vi "PSK_Mod_Transmit_test_Q.vi"() -> ()   [LabVIEW 2014]
uses:
  <vilib>/addons/Modulation/Analog/controls/Complex Data Waveform.ctl
  <vilib>/addons/Modulation/Digital/General/MT Generate Bits (Galois, PN Order).vi
  <vilib>/addons/Modulation/Digital/Support/Common/Validators/mod_Generate Bits Validate.vi
  <vilib>/addons/Modulation/Analog/support/mod_Set Error Source.vi
  <vilib>/addons/Modulation/Digital/General/subVIs/mod_Generate Bits PN Sequence.vi
  <instrlib>/niUSRP/niUSRP Write Tx Data (CDB Cluster).vi
  <vilib>/addons/Modulation/niDMT.lvlib
  <vilib>/addons/Modulation/niAMT.lvlib
panel:
  out "Antall pakker generert":i32
  out "# elements in queue 1":i32
  out "# elements in queue 2":i32
  out "Antall pakker faktisk sendt":dbl
  out "Number of message bits in burst":i32
  out "After mod":waveform(dbl)(graph)
  out "Tid pakkegen":dbl
  out "Tid modulator":dbl
  out "Tid Sender":dbl
  in  "stop":bool
  in  "Packet Parameters":T1={"Length of sync sequence (20)"=30, "Number of message bits"=128, "Number of guardbits"=40, "PN sequence order (31)"=31, "Number of packets in burst"=30}
  out "Constellation Graph":T2(graph) caption="Tx Signal Constellation"
  out "bits pr burst":i32
  out "input bit stream":i8[](array[numeric]) caption="input package"
  out "time/packet":dbl
  out "error out":errorcluster
  in  "USRP IP address":refnum<k15>="192.168.10.1"
  in  "Tx Parameters":T3={"Tx IQ Sampling\nRate [s/sec]"=400000.0, "Tx Frequency [Hz]"=5795000000.0, "Tx Gain [dB]"=10.0, "Tx Antenna"="TX1"} {"Tx Gain [dB]" format="%#.6p"; "Tx Frequency [Hz]" format="%#.6p"; "Tx IQ Sampling\nRate [s/sec]" format="%#.6p"}
  out "Actual Tx Parameters":T3={"Tx IQ Sampling\nRate [s/sec]"=400000.0, "Tx Frequency [Hz]"=915000000.0, "Tx Gain [dB]"=0.0, "Tx Antenna"="TX1"} {"Tx Gain [dB]" format="%#.6p"; "Tx Frequency [Hz]" format="%#.6p"; "Tx IQ Sampling\nRate [s/sec]" format="%#.6p"}
  in  "filter parameters":T4={"Alpha"=0.5, "Filter Length"=6, "TX Filter"=enum."Root Raised Cos"} {"Alpha" format="%.2f"}
  in  "QPSK System Parameters":T5={"Samples per Symbol"=8, "symbol map"=[], "Differential PSK"=enum."disable", "PSK type"=0, "M-PSK (4)"=4} {"PSK type" items=["normal", "shifted", "offset"]; "symbol map" format="%.3f"}
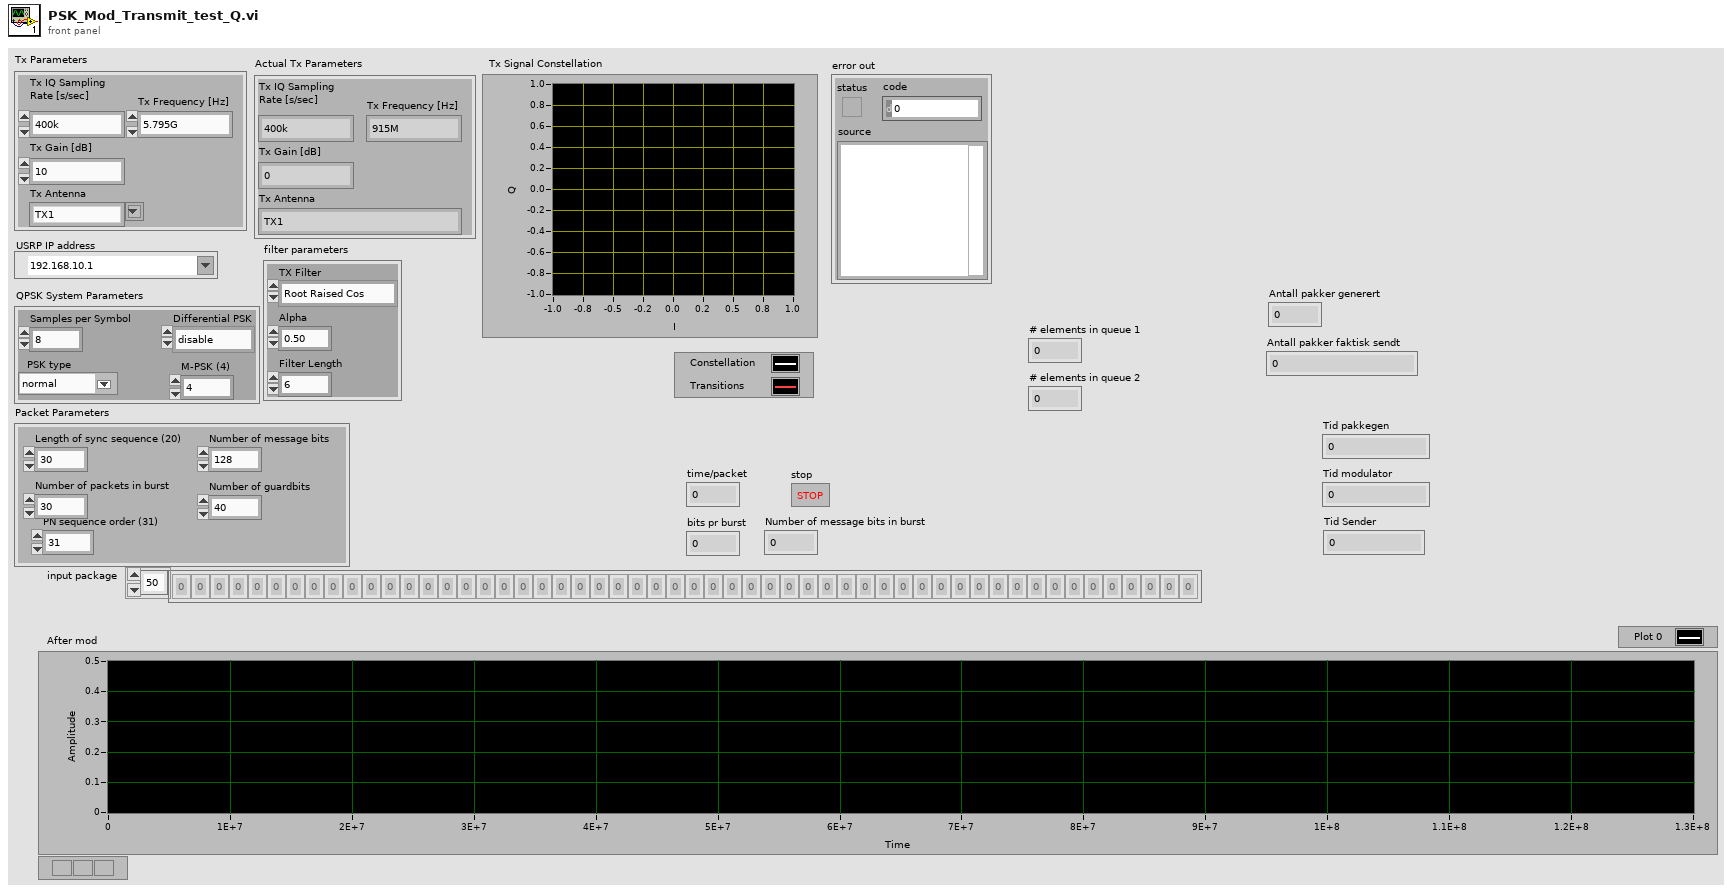
[diagram p1: front panel]
types:
  T1 = cluster{"Length of sync sequence (20)":i32, "Number of message bits":i32, "Number of guardbits":i32, "PN sequence order (31)":i32, "Number of packets in burst":i32}
  T2 = cluster{"constellation":dbl[], "oversampled data":dbl[]}[]
  T3 = cluster{"Tx IQ Sampling\nRate [s/sec]":dbl, "Tx Frequency [Hz]":dbl, "Tx Gain [dB]":dbl, "Tx Antenna":string}
  T4 = cluster{"Alpha":dbl, "Filter Length":i32, "TX Filter":enum16{"none", "Raised Cosine", "Root Raised Cos", "Gaussian"}}
  T5 = cluster{"Samples per Symbol":i32, "symbol map":cdb[], "Differential PSK":enum16{"disable", "enable"}, "PSK type":u16, "M-PSK (4)":i32}
  T6 = typedef "niAMT.lvlib/Complex Data Waveform.ctl" = cluster{"t0":dbl, "dt":dbl, "Y":cdb[]}
  T7 = cluster{"samples per symbol (16)":i32, "symbol map":cdb[], "differential PSK":enum16{"disable", "enable"}, "PSK type":u16}
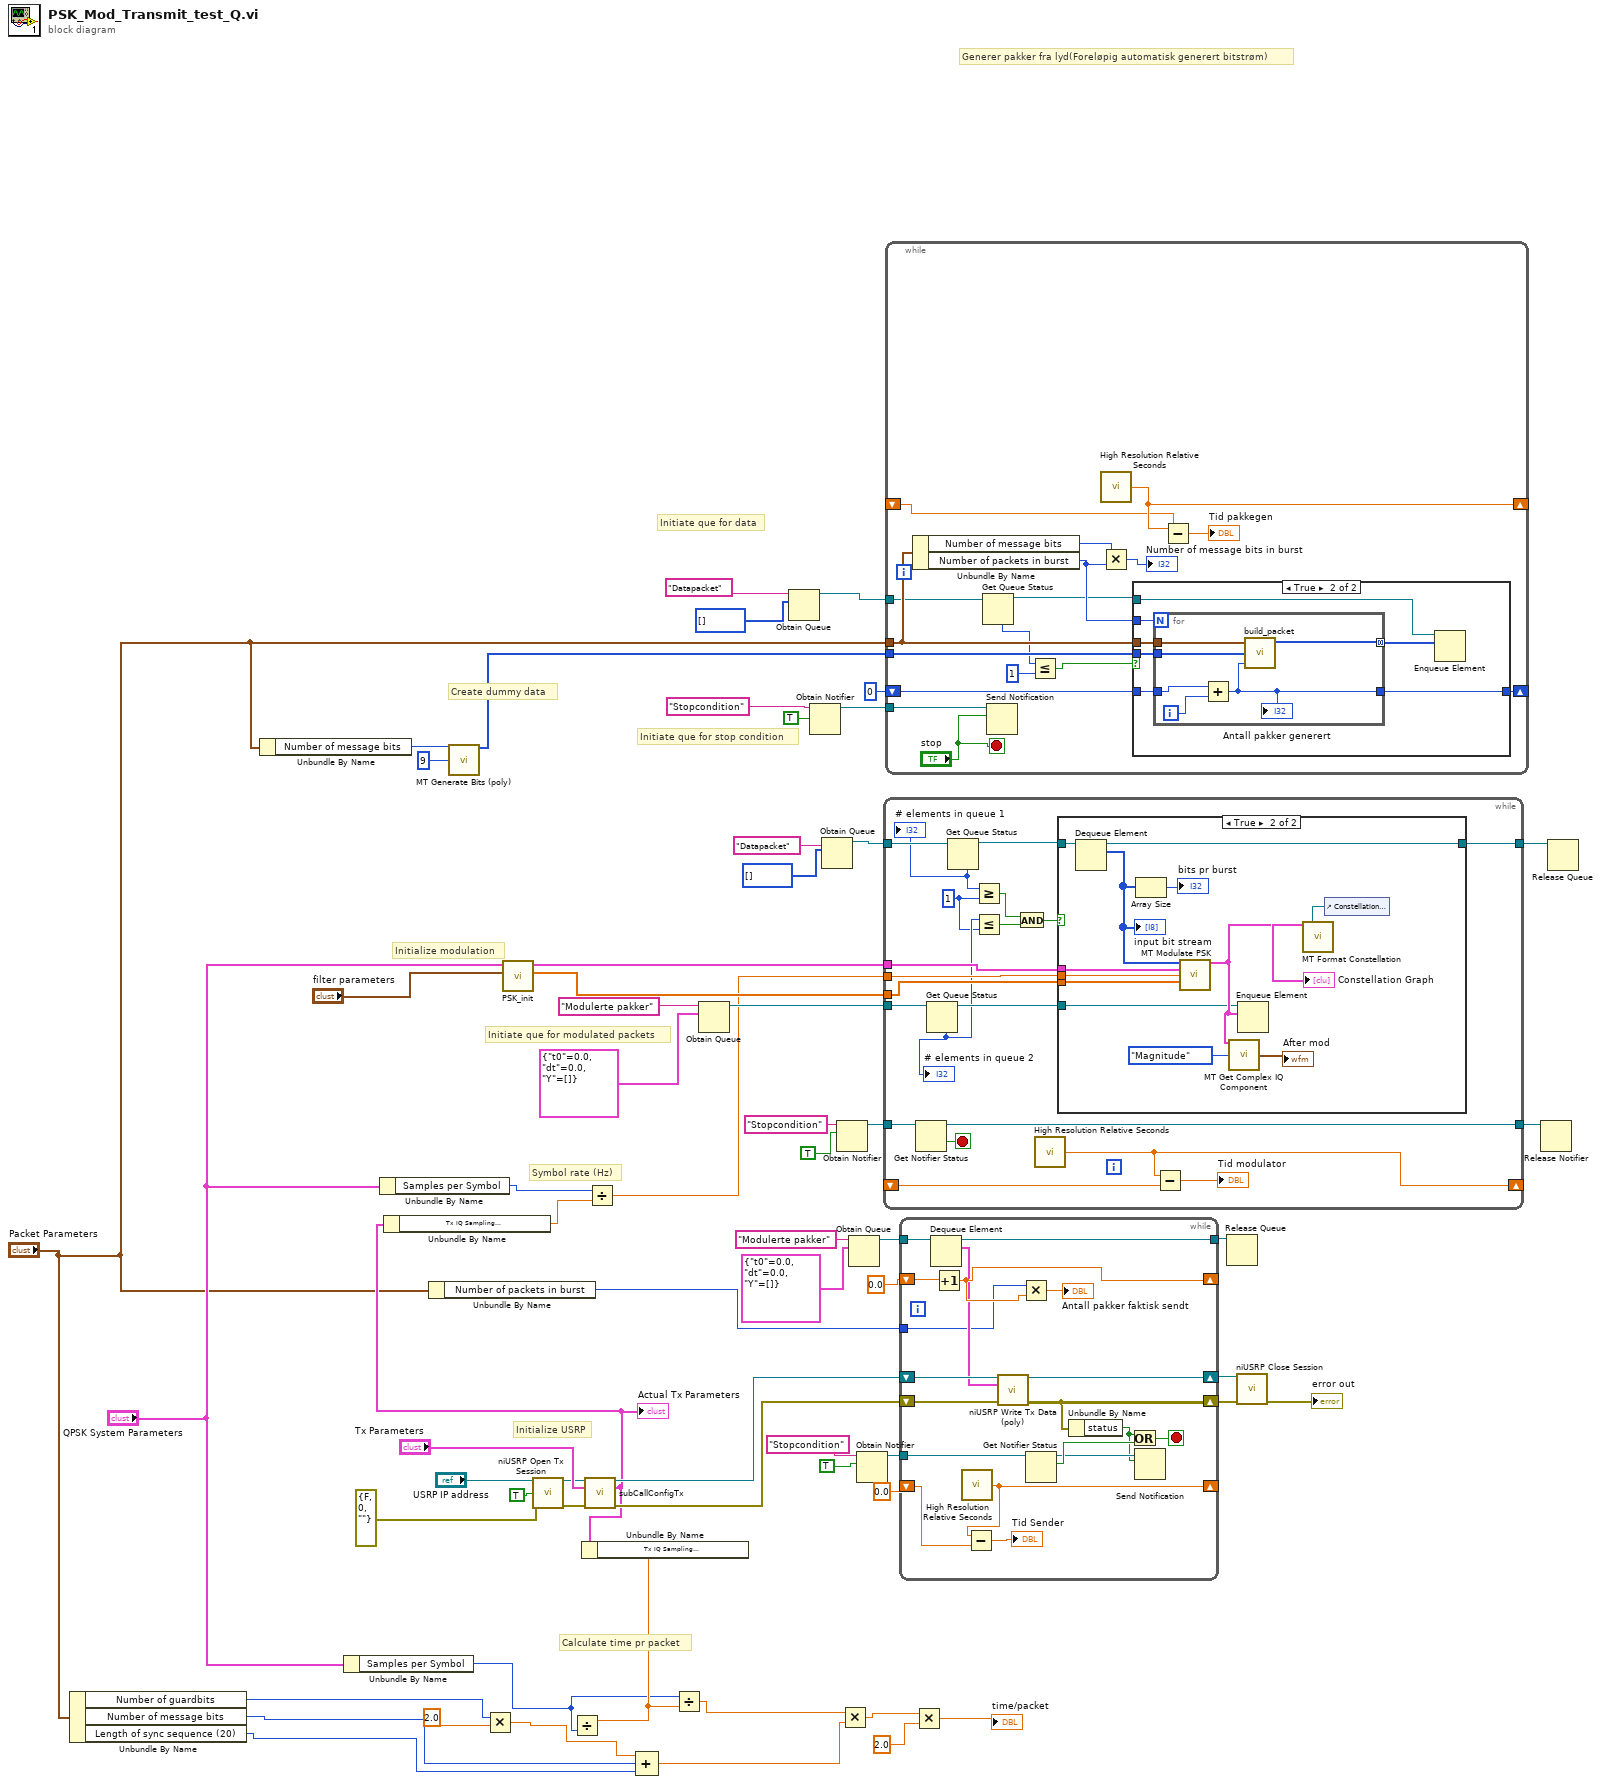
[diagram p0: block diagram]
diagram:
  # "Calculate time pr packet"
  # "Initialize USRP"
  # "Initialize modulation"
  # "Initiate que for modulated packets"
  # "Create dummy data"
  # "Initiate que for stop condition"
  # "Initiate que for data"
  # "Generer pakker fra lyd(Foreløpig automatisk generert bitstrøm)"
  # "Symbol rate (Hz)"
  n1 = Unbundle By Name("Packet Parameters") -> ("Number of guardbits"=w46:i32, "Number of message bits"=w40:i32, "Length of sync sequence (20)"=w44:i32)
  n2 = Unbundle By Name("Packet Parameters") -> ("Number of message bits"=w18:i32)
  n3 = Unbundle By Name("QPSK System Parameters") -> ("Samples per Symbol"=w43:i32)
  n4 = Unbundle By Name("QPSK System Parameters") -> ("Samples per Symbol"=w25:i32)
  n5 = Unbundle By Name("Packet Parameters") -> ("Number of packets in burst"=w2:i32)
  n6 = call-poly <vilib>:"MT Generate Bits (poly).vi"("total bits (128)"=w18, "PN sequence order (9)"=9) -> ("output bit stream"=w19:i8[])  [unwired: 11 in, 2 out]
  n7 = Multiply(x=w46, y=2.0 ("x")) -> (x*y=w53:dbl)
  n8 = call "PSK_init.vi"("filter parameters"="filter parameters", "QPSK System Parameters"="QPSK System Parameters") -> ("matched filter coefficients"=w27:dbl[], "PSK system parameters"=w28:T7)  [unwired: 5 in, 2 out]
  n9 = call <instrlib>:"niUSRP Open Tx Session.vi"("device names"="USRP IP address", "reset"=TRUE, "error in (no error)"=errorcluster {"status"=FALSE, "code"=0, "source"=""}) -> ("session handle out"=w62:refnum<k15>, "error out"=w61:errorcluster)  [unwired: 11 in]
  n10 = call "subCallConfigTx.vi"("session handle"=w62, "Tx Parameters"="Tx Parameters", "error in"=w61) -> ("session handle out"=w57:refnum<k15>, "Actual Tx Parameters"=w21:T3, "error out"=w35:errorcluster)  [unwired: 10 in]
  "Actual Tx Parameters" <- w21
  n11 = Unbundle By Name(w21) -> ("Tx IQ Sampling\nRate [s/sec]"=w24:dbl)
  n12 = Unbundle By Name(w21) -> ("Tx IQ Sampling\nRate [s/sec]"=w52:dbl)
  n13 = Divide(x=w52, y=w43) -> ()  [unwired: 1 out]
  n14 = Divide(x=w25, y=w24) -> (x/y=w23:dbl)
  n15 = Compound Arithmetic op=ADD(w53, w40, w44) -> (w50:dbl)
  n16 = Divide(x=w43, y=w52) -> (x/y=w51:dbl)
  n17 = Obtain Queue(name (unnamed)="Modulerte pakker", element data type=T6 {"t0"=0.0, "dt"=0.0, "Y"=[]} ("output complex waveform")) -> (queue out=w31:refnum<queue>)  [unwired: 3 in, 2 out]
  n18 = Obtain Queue(name (unnamed)="Datapacket", element data type=i8[] [] ("output bitstream")) -> (queue out=w37:refnum<queue>)  [unwired: 3 in, 2 out]
  n19 = Obtain Notifier(name (unnamed)="Stopcondition", notification data type=TRUE ("stop 2")) -> (notifier out=w34:refnum<notifier>)  [unwired: 2 in, 2 out]
  n20 = Obtain Queue(name (unnamed)="Datapacket", element data type=i8[] [] ("output bitstream")) -> (queue out=w11:refnum<queue>)  [unwired: 3 in, 2 out]
  n21 = Obtain Notifier(name (unnamed)="Stopcondition", notification data type=TRUE ("stop 2")) -> (notifier out=w14:refnum<notifier>)  [unwired: 2 in, 2 out]
  n22 = Multiply(x=w51, y=w50) -> (x*y=w48:dbl)
  n23 = Obtain Queue(name (unnamed)="Modulerte pakker", element data type=T6 {"t0"=0.0, "dt"=0.0, "Y"=[]} ("output complex waveform")) -> (queue out=w17:refnum<queue>)  [unwired: 3 in, 2 out]
  n24 = Obtain Notifier(name (unnamed)="Stopcondition", notification data type=TRUE ("stop 2")) -> (notifier out=w13:refnum<notifier>)  [unwired: 2 in, 2 out]
  n25 = while {
    tunnel: w11 -> [w74]
    tunnel: [w83] -> w36
    tunnel: w27 -> [w82]
    tunnel: w28 -> [w81]
    tunnel: w23 -> [w80]
    tunnel: w14 -> [w79]
    tunnel: w31 -> [w75]
    shift-right: [w76] -> _
    shift-left: _ -> [w77]
    tunnel: [w64] -> w1
    stop <- w78 stop-if-true
    w67 = 1 ("y")
    n26 = Get Notifier Status(notifier=w79) -> (notifier out=w64:refnum<notifier>, current notification=w78:bool)  [unwired: 1 in, 3 out]
    n27 = Get Queue Status(queue=w75) -> (queue out=w72:refnum<queue>, # elements in queue=w71:i32)  [unwired: 2 in, 6 out]
    "# elements in queue 2" <- w71
    n28 = Get Queue Status(queue=w74) -> (queue out=w73:refnum<queue>, # elements in queue=w68:i32)  [unwired: 2 in, 6 out]
    "# elements in queue 1" <- w68
    n29 = Greater Or Equal?(x=w68, y=w67) -> (x >= y?=w69:bool)
    n30 = Less Or Equal?(x=w71, y=w67) -> (x <= y?=w70:bool)
    n31 = And(x=w69, y=w70) -> (x .and. y?=w66:bool)
    n32 = call <vilib>:"High Resolution Relative Seconds.vi"() -> ("relative seconds"=w76:dbl)
    n33 = case shown="True" w66 {
      tunnel: w73 -> [w84 w97]
      tunnel: [w84 w96] -> w83
      tunnel: w82 -> [_ w92]
      tunnel: w81 -> [_ w91]
      tunnel: w80 -> [_ w90]
      tunnel: w72 -> [_ w85]
      frame False {
      }
      frame True {
        n34 = Dequeue Element(queue=w97) -> (queue out=w96:refnum<queue>, element=w89:i8[])  [unwired: 2 in, 2 out]
        "input bit stream" <- w89
        n35 = Array Size(array=w89) -> (size(s)=→"bits pr burst":i32)
        n36 = call <vilib>:"MT Modulate PSK.vi"("input bit stream"=w89, "PSK system parameters"=w91, "symbol rate (Hz)"=w90, "pulse shaping filter coefficients"=w92) -> ("output complex waveform"=w86:T6)  [unwired: 9 in, 2 out]
        n37 = call <vilib>:"MT Get Complex IQ Component.vi"("IQ data (complex) in"=w86, "component choice"=enum16{"I", "Q", "Magnitude", "Phase"}."Magnitude") -> ("CE component"=→"After mod":waveform(dbl))  [unwired: 11 in, 2 out]
        n38 = Enqueue Element(queue=w85, element=w86) -> ()  [unwired: 2 in, 3 out]
        n39 = control-ref of="Constellation Graph"() -> (w93:refnum<vi>)
        n40 = call <vilib>:"MT Format Constellation.vi"("waveform"=w86, "constellation reference"=w93) -> ("constellation graph"=→"Constellation Graph":T2)  [unwired: 12 in, 1 out]
      }
    }
    n41 = Subtract(x=w76, y=w77) -> (x-y=→"Tid modulator":dbl)
  }
  n42 = while {
    tunnel: "Packet Parameters" -> [w110]
    tunnel: w19 -> [w113]
    tunnel: w37 -> [w106]
    tunnel: w34 -> [w114]
    shift-right: [w112] -> _
    shift-left: _ -> [w111]
    shift-right: [w98] -> _
    shift-left: 0 -> [w99]
    stop <- "stop" stop-if-true
    n43 = Unbundle By Name(w110) -> ("Number of message bits"=w109:i32, "Number of packets in burst"=w107:i32)
    n44 = Get Queue Status(queue=w106) -> (queue out=w105:refnum<queue>, # elements in queue=w104:i32)  [unwired: 2 in, 6 out]
    n45 = Send Notification(notification="stop", notifier=w114) -> ()  [unwired: 1 in, 2 out]
    n46 = Less Or Equal?(x=w104, y=1) -> (x <= y?=w103:bool)
    n47 = call <vilib>:"High Resolution Relative Seconds.vi"() -> ("relative seconds"=w112:dbl)
    n48 = Multiply(x=w109, y=w107) -> (x*y=→"Number of message bits in burst":i32)
    n49 = case shown="True" w103 {
      tunnel: w105 -> [_ w122]
      tunnel: w113 -> [_ w121]
      tunnel: w110 -> [_ w119]
      tunnel: w107 -> [_ w118]
      tunnel: w99 -> [w115 w117]
      tunnel: [w115 w116] -> w98
      frame False {
      }
      frame True {
        n50 = for {
          N: w118 -> [_]
          tunnel: w121 -> [w128]
          tunnel: w119 -> [w127]
          tunnel: [w126] -> w120 mode=concatenating
          tunnel: w117 -> [w123]
          tunnel: [w124] -> w116
          i -> [w125]
          n51 = Add(x=w123, y=w125) -> (x+y=w124:i32)
          "Antall pakker generert" <- w124
          n52 = call "build_packet.vi"("Packet number"=w124, "message data"=w128, "Packet Parameters"=w127) -> ("output bitstream"=w126:i8[])  [unwired: 5 in]
        }
        n53 = Enqueue Element(queue=w122, element=w120) -> ()  [unwired: 2 in, 3 out]
      }
    }
    n54 = Subtract(x=w112, y=w111) -> (x-y=→"Tid pakkegen":dbl)
  }
  n55 = while {
    shift-right: [w136] -> w55
    shift-left: w35 -> [w139]
    shift-right: [w137] -> w56
    shift-left: w57 -> [w138]
    tunnel: w13 -> [w146]
    tunnel: [w140] -> w30
    shift-right: [w144] -> _
    shift-left: 0.0 ("relative seconds") -> [w145]
    shift-right: [w134] -> _
    shift-left: 0.0 -> [w135]
    tunnel: w17 -> [w141]
    tunnel: w2 -> [w131]
    stop <- w147 stop-if-true
    n56 = Dequeue Element(queue=w141) -> (queue out=w140:refnum<queue>, element=w133:T6)  [unwired: 2 in, 2 out]
    n57 = Increment(x=w135) -> (x+1=w134:dbl)
    n58 = call <vilib>:"High Resolution Relative Seconds.vi"() -> ("relative seconds"=w144:dbl)
    n59 = Subtract(x=w144, y=w145) -> (x-y=→"Tid Sender":dbl)
    n60 = call-poly <instrlib>:"niUSRP Write Tx Data (poly).vi"("session handle"=w138, "data"=w133, "error in (no error)"=w139) -> ("session handle out"=w137:refnum<k15>, "error out"=w136:errorcluster)  [unwired: 11 in]
    n61 = Multiply(x=w131, y=w134) -> (x*y=→"Antall pakker faktisk sendt":dbl)
    n62 = Get Notifier Status(notifier=w146) -> (notifier out=w130:refnum<notifier>, current notification=w132:bool)  [unwired: 1 in, 3 out]
    n63 = Unbundle By Name(w136) -> ("status"=w129:bool)
    n64 = Or(x=w129, y=w132) -> (x .or. y?=w147:bool)
    n65 = Send Notification(notification=w129, notifier=w130) -> ()  [unwired: 1 in, 2 out]
  }
  n66 = Multiply(x=w48, y=2.0) -> (x*y=→"time/packet":dbl)
  n67 = Release Queue(queue=w30) -> ()  [unwired: 2 in, 3 out]
  n68 = call <instrlib>:"niUSRP Close Session.vi"("session handle"=w56, "error in (no error)"=w55) -> ("error out"=→"error out":errorcluster)  [unwired: 13 in]
  n69 = Release Notifier(notifier=w1) -> ()  [unwired: 2 in, 3 out]
  n70 = Release Queue(queue=w36) -> ()  [unwired: 2 in, 3 out]
